vi "SendDataToAllClients.vi"(8 "error in (no error)":errorcluster, 9 "data":variant, 10 "ServerActions":T1, 11 "Gserver in":refnum<class "Gserver.lvclass">) -> (0 "error out":errorcluster, 3 "Gserver out":refnum<class "Gserver.lvclass">)   [LabVIEW 2020, in "Sgraph_lib_V1.lvlib" / "Gserver.lvclass"]
doc: "Andre Koelewijn, 5 jan 2021\n\nSend data to all active Vgraph Clients"
uses:
  Gserver.lvclass
  Gview/controls/Typedef_ServerActions.ctl
  Gserver.lvclass/Gserver.ctl
  Gview/controls/Typedef_Gserver-Replies.ctl
  Gview/Gviewer.lvclass
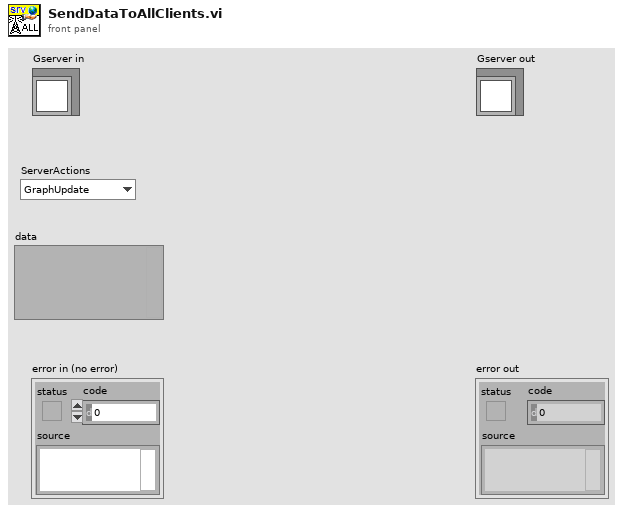
[diagram p1: front panel]
types:
  T1 = typedef "Sgraph_lib_V1.lvlib/Gviewer.lvclass/Typedef_ServerActions.ctl" = enum16{"GraphUpdate", "SendAllTags", "SendIniPath", "SetGeneralOptions", "EditTagsOpen", "EditTagsPresetSave", "EditTagsPresetLoad", "EditTagsClose", "NewTagSelection", "AutoScale", "DBeditStatus", "DBsaveConfirm", "GetXconstraints", "ExitGraph"}
  T2 = typedef "Typedef_Gserver-Replies.ctl" = cluster{"ServerActions":T1, "data":variant, "Source":string, "Time Stamp":timestamp}
  T3 = typedef "Sgraph_lib_V1.lvlib/Gserver.lvclass/Typedef_Sgraph_Query.ctl" = cluster{"ViewportName":string, "Tags":string[], "Time-Start":timestamp, "Time-End":timestamp, "Pixels":i32, "Live":T4, "TimeSpan(sec)":dbl, "GViewer-Queue":refnum<queue>}
  T4 = typedef "Sgraph_lib_V1.lvlib/Gviewer.lvclass/Typedef_Live.ctl" = enum16{"Live View", "Freeze"}
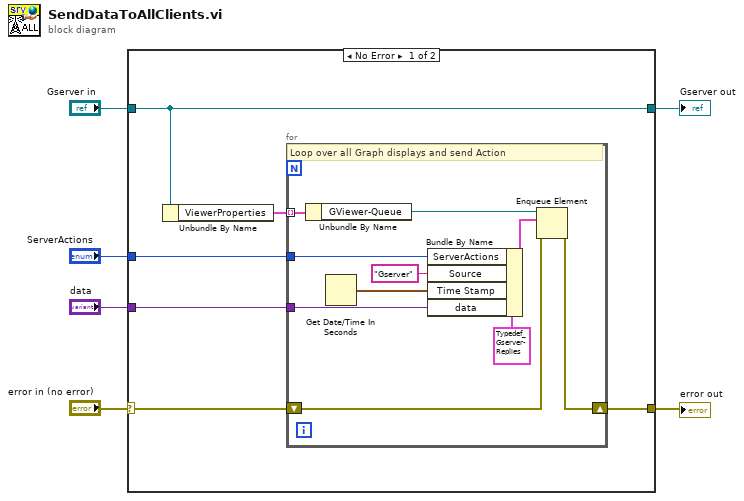
[diagram p0: block diagram]
diagram:
  n1 = case shown="No Error" "error in (no error)" {
    selector: "error in (no error)" -> [w10 w24]
    tunnel: [w9 w24] -> w5
    tunnel: [w11 w23] -> w3
    tunnel: "Gserver in" -> [w11 w23]
    tunnel: "ServerActions" -> [w8 _]
    tunnel: "data" -> [w7 _]
    frame No Error {
      n2 = Unbundle By Name(w11) -> ("ViewerProperties"=w12:T3[])
      n3 = for {
        tunnel: w12 -> [w22] mode=indexing
        shift-right: [w19] -> w9
        shift-left: w10 -> [w20]
        tunnel: w8 -> [w14]
        tunnel: w7 -> [w13]
        # "Loop over all Graph displays and send Action"
        n4 = Unbundle By Name(w22) -> ("GViewer-Queue"=w21:refnum<queue>)
        n5 = Get Date/Time In Seconds() -> (seconds since 1Jan1904=w15:timestamp)
        n6 = Bundle By Name(cluster=T2 {"ServerActions"=enum."GraphUpdate", "data"=variant, "Source"="", "Time Stamp"=timestamp(0 s since 1904-01-01)} ("element"), "ServerActions"=w14, "Source"="Gserver", "Time Stamp"=w15, "data"=w13) -> (w17:T2)
        n7 = Enqueue Element(queue=w21, element=w17, error in (no error)=w20) -> (error out=w19:errorcluster)  [unwired: 1 in, 2 out]
      }
    }
    frame Error {
    }
  }
  "error out" <- w5
  "Gserver out" <- w3
